vi "Get Command Bits Field Width.vi"(8 "error in (no error)":errorcluster, 11 "RFFE Command in":refnum<class "RFFE Command.lvclass">) -> (0 "error out":errorcluster, 2 "Command Bits Field Width":i32, 3 "RFFE Command out":refnum<class "RFFE Command.lvclass">)   [LabVIEW 2018, in "MIPI RFFE API.lvlib" / "RFFE Command.lvclass"]
uses:
  RFFE Command.lvclass
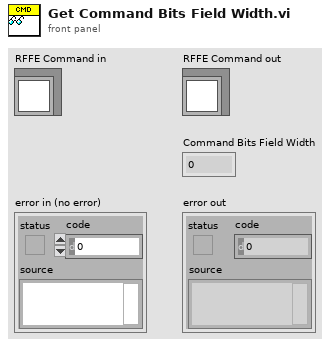
[diagram p1: front panel]
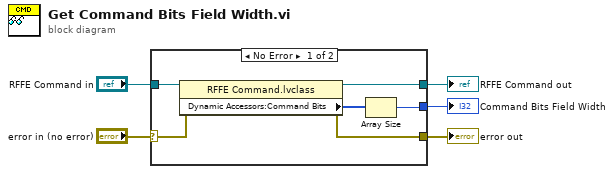
[diagram p0: block diagram]
diagram:
  n1 = case shown="No Error" "error in (no error)" {
    selector: "error in (no error)" -> [w8 w12]
    tunnel: [w9 w12] -> w4
    tunnel: [w11 w13] -> w2
    tunnel: "RFFE Command in" -> [w10 w13]
    tunnel: [w6 _] -> w1
    frame No Error {
      n2 = property class="RFFE Command.lvclass"(reference=w10, error in=w8) -> (reference out=w11:refnum<class "RFFE Command.lvclass">, error out=w9:errorcluster, "Dynamic Accessors:Command Bits"=w7:u8[])
      n3 = Array Size(array=w7) -> (size(s)=w6:i32)
    }
    frame Error {
    }
  }
  "error out" <- w4
  "RFFE Command out" <- w2
  "Command Bits Field Width" <- w1
